vi "Log Error.vi"(9 "Source":string, 11 "error in":errorcluster) -> (3 "error out":errorcluster)   [LabVIEW 2014]
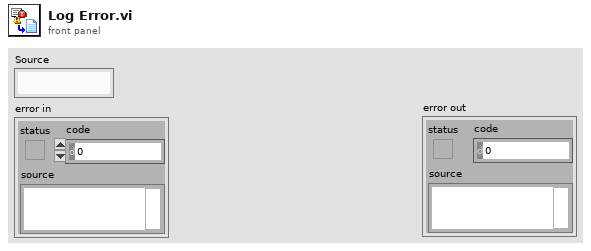
[diagram p1: front panel]
types:
  T1 = enum16{"open", "replace", "create", "open or create", "replace or create", "replace or create with confirmation"}
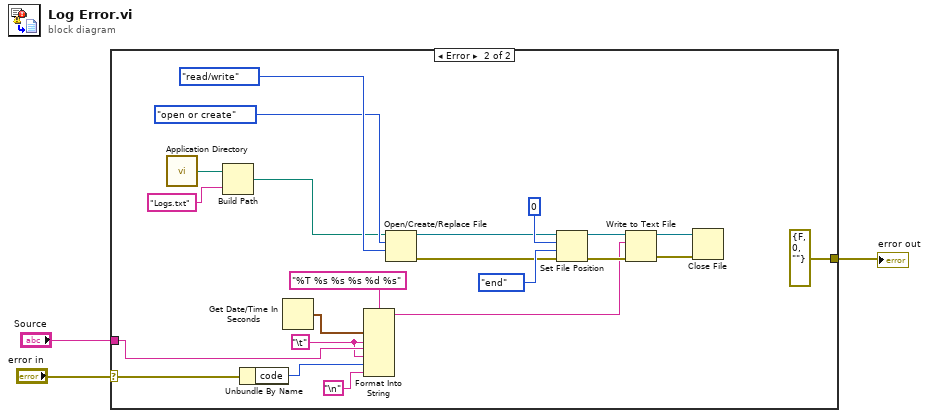
[diagram p0: block diagram]
diagram:
  n1 = case shown="Error" "error in" {
    selector: "error in" -> [w4 w22]
    tunnel: [w4 errorcluster {"status"=FALSE, "code"=0, "source"=""} ("error constant")] -> w3
    tunnel: "Source" -> [_ w12]
    frame No Error {
    }
    frame Error {
      w11 = "\t"
      n2 = call <vilib>:"Application Directory.vi"() -> ("Application Directory"=w17:path)
      n3 = Build Path(base path=w17, name or relative path="Logs.txt") -> (appended path=w18:path)
      n4 = Unbundle By Name(w22) -> ("code"=w10:i32)
      n5 = Get Date/Time In Seconds() -> (seconds since 1Jan1904=w21:timestamp)
      n6 = Format Into String(format string="%T %s %s %s %d %s", w21, w11, w12, w11, w10, "\n") -> (resulting string=w13:string)  [unwired: 2 in, 1 out]
      n7 = Open/Create/Replace File(file path (use dialog)=w18, operation (0:open)=T1."open or create", access (0:read/write)=enum16{"read/write", "read-only", "write-only"}."read/write") -> (refnum out=w15:refnum<file>, error out=w5:errorcluster)  [unwired: 3 in, 1 out]
      n8 = Set File Position(offset (in bytes) (0)=i64 0, refnum=w15, from (0:start)=enum16{"start", "end", "current"}."end", error in=w5) -> (refnum out=w25:refnum<file>, error out=w26:errorcluster)
      n9 = Write to Text File(file (use dialog)=w25, text=w13, error in=w26) -> (refnum out=w7:refnum<file>, error out=w6:errorcluster)  [unwired: 1 in, 1 out]
      n10 = Close File(refnum=w7, error in=w6) -> ()  [unwired: 2 out]
    }
  }
  "error out" <- w3
